vi "全局1.vi"() -> ()   [LabVIEW 2020]
panel:
  in  "左加载":dbl
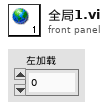
[diagram p1: front panel]
diagram:
